vi "DIGITAL TDMS.vi"(8 "DIGITAL DAQ 2":bool[](array[boolean]), 11 "NAME":string) -> ()   [LabVIEW 2020, in "Logging.lvlib"]
uses:
  Logging.lvlib
  <vilib>/Utility/sysdir.llb/System Directory Type.ctl
  <vilib>/Utility/TDMS File Viewer/NI_TDMS File Viewer.lvlib
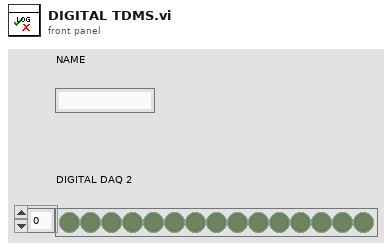
[diagram p1: front panel]
types:
  T1 = enum16{"open", "open or create", "create or replace", "create", "open (read-only)"}
  T2 = typedef "System Directory Type.ctl" = i32
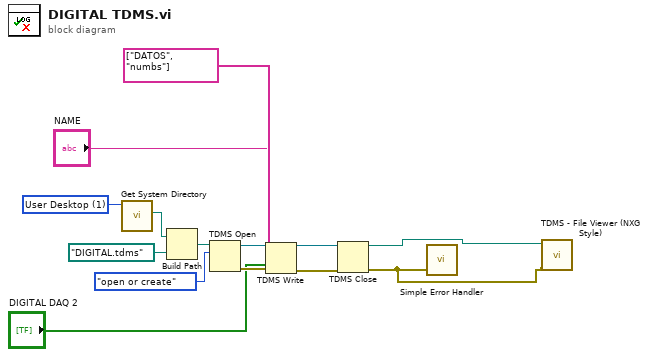
[diagram p0: block diagram]
diagram:
  w13 = T2 1 items=["User Home"=0, "User Desktop"=1, "User Documents"=2, "User Application Data"=3, "User Preferences"=4, "User Temporary"=5, "Public Documents"=6, "Public Application Data"=7, "Public Preferences"=8, "Public Cache"=13, "System Core Libraries"=9, "System Installed Libraries"=10, "Application Files"=11, "Boot Volume Root"=12] ("system directory type")
  n1 = call <vilib>:"Get System Directory.vi"("system directory type"=w13) -> ("system directory"=w14:path)  [unwired: 10 in]
  n2 = Build Path(base path=w14, name or relative path=path "DIGITAL.tdms") -> (appended path=w11:path)
  n3 = TDMS Open(10:T1."open or create" ("operation (0:open)"), 11:w11) -> (0:w7:errorcluster, 3:w9:refnum<k34>)  [unwired: 5 in]
  n4 = TDMS Write(0:w9, 5:"NAME", 7:string[] ["DATOS", "numbs"] ("channel name(s) in (Untitled)"), 9:"DIGITAL DAQ 2", 11:w7) -> (4:w8:refnum<k34>, 15:w6:errorcluster)  [unwired: 1 in, 2 out]
  n5 = TDMS Close(8:w6, 11:w8) -> (0:w3:errorcluster, 3:w4:path)
  n6 = call <vilib>:"Simple Error Handler.vi"("error in (no error)"=w3) -> ()  [unwired: 4 in, 5 out]
  n7 = call <vilib>:"TDMS - File Viewer (NXG Style).vi"("error in"=w3, "file in"=w4) -> ()  [unwired: 8 in, 2 out]
